vi "Write DIO mode.vi"(8 "error in (no error)":errorcluster, 10 "DIO mode":u32(ring) items=["Normal", "Counter", "Counter Slave", "PWM", "Quadrature"], 11 "SD Module in":refnum<class "SD Module.lvclass">) -> (0 "error out":errorcluster, 3 "SD Module out":refnum<class "SD Module.lvclass">)   [LabVIEW 2019, in "Modules.lvlib" / "SD Module.lvclass"]
uses:
  SD Module.lvclass
  SD Module.lvclass/SD Module.ctl
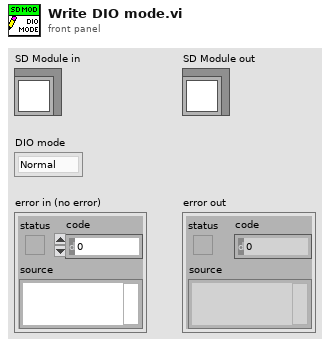
[diagram p1: front panel]
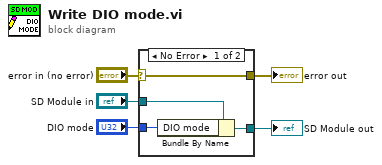
[diagram p0: block diagram]
diagram:
  n1 = case shown="No Error" "error in (no error)" {
    selector: "error in (no error)" -> [w9 w10]
    tunnel: [w9 w10] -> w4
    tunnel: [w7 w11] -> w2
    tunnel: "SD Module in" -> [w8 w11]
    tunnel: "DIO mode" -> [w6 _]
    frame No Error {
      n2 = Bundle By Name(cluster=w8, "DIO mode"=w6) -> (w7:refnum<class "SD Module.lvclass">)
    }
    frame Error {
    }
  }
  "error out" <- w4
  "SD Module out" <- w2
